vi "UDT__loggingModule_sendErrorLog.vi"() -> (3 "Unit Test Framework Results":T1)   [LabVIEW 2017]
doc: "Use this template to create a user-defined test VI. Define your test requirements and wire the results to the <b>Result (Test)</b> control. Do not modify the <b>Unit Test Framework Results</b> indicator."
uses:
  <vilib>/utf/common/utf_test_result_troll.ctl
  <vilib>/utf/common/utf_test_result.ctl
  <vilib>/utf/common/utf_test_result_failure.ctl
  <vilib>/utf/common/utf_test_comparison_operators.ctl
  <vilib>/utf/common/utf_vi_tag.ctl
  RT/loggingModule/Queue/TypeDefs/queueFGVState.ctl
  RT/ErrorMonitor/Queue/TypeDefs/message.ctl
  RT/loggingModule/loggingModule.lvlib
  <vilib>/Control Software Solutions Ltd/UTF Helper/Unit Test Helper.lvlib
  RT/ErrorMonitor/ErrorMonitor.lvlib
  <vilib>/utf/NI_UnitTestFramework.lvlib
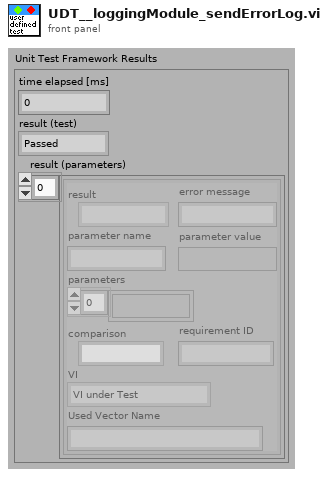
[diagram p1: front panel]
types:
  T1 = typedef "NI_UnitTestFramework.lvlib/utf_test_result_troll.ctl" = cluster{"time elapsed [ms]":u32, "result (test)":T2, "result (parameters)":T3[]}
  T2 = typedef "NI_UnitTestFramework.lvlib/utf_test_result.ctl" = enum16{"Passed", "Failed", "Error", "Skipped", "Not Processed"}
  T3 = typedef "NI_UnitTestFramework.lvlib/utf_test_result_failure.ctl" = cluster{"result":T2, "error message":string, "parameter name":string, "parameter value":variant, "parameters":variant[], "comparison":T4, "requirement ID":string, "VI":T5, "Used Vector Name":string}
  T4 = typedef "NI_UnitTestFramework.lvlib/utf_test_comparison_operators.ctl" = enum16{"=", "!=", ">", ">=", "<", "<=", "range", "symmetric tolerance", "asymmetric tolerance", "string contains", "string not contain", "array size", "string length", "array range", "by element", "array range (limit array)", "user-defined", "array contains", "array not contain", "vector length", "= (elm)", "!= (elm)", "= (case insensitive)", "!= (case insensitive)"}
  T5 = typedef "NI_UnitTestFramework.lvlib/utf_vi_tag.ctl" = enum16{"Setup VI", "VI under Test", "Teardown VI"}
  T6 = typedef "ErrorMonitor.lvlib/message.ctl" = cluster{"calling module":string, "message":string, "Data":variant}
  T7 = typedef "loggingModule.lvlib/queueFGVState.ctl" = enum16{"obtain", "enqueue low priority", "enqueue high priority", "dequeue", "release"}
  T8 = typedef "loggingModule.lvlib/message.ctl" = cluster{"calling module":string, "message":string, "data":variant}
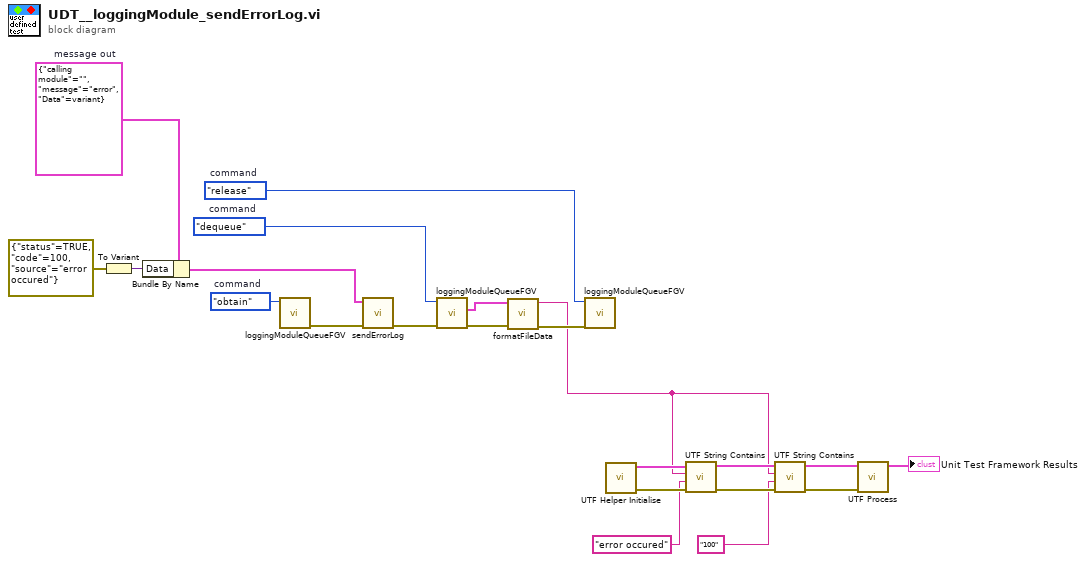
[diagram p0: block diagram]
diagram:
  w4 = T6 {"calling module"="", "message"="error", "Data"=variant}  # message out
  w20 = queueFGVState."release"  # command
  w21 = queueFGVState."dequeue"  # command
  w22 = queueFGVState."obtain"  # command
  n1 = To Variant(anything=errorcluster {"status"=TRUE, "code"=100, "source"="error occured"} ("error constant")) -> (Variant=w1:variant)
  n2 = Bundle By Name(cluster=w4, "Data"=w1) -> (w3:T6)
  n3 = call "loggingModuleQueueFGV.vi"("command"=w22) -> ("error out"=w6:errorcluster)  [unwired: 9 in, 1 out]
  n4 = call "sendErrorLog.vi"("error in (no error)"=w6, "message out"=w3) -> ("error out"=w5:errorcluster)  [unwired: 9 in]
  n5 = call "loggingModuleQueueFGV.vi"("error in (no error)"=w5, "command"=w21) -> ("error out"=w13:errorcluster, "message out"=w11:T8)  [unwired: 8 in]
  n6 = call "formatFileData.vi"("error in (no error)"=w13, "message out"=w11) -> ("error out"=w12:errorcluster, "LogData"=w10:string)  [unwired: 8 in]
  n7 = call "loggingModuleQueueFGV.vi"("error in (no error)"=w12, "command"=w20) -> ()  [unwired: 8 in, 2 out]
  n8 = call <vilib>:"UTF Helper Initialise.vi"() -> ("error out"=w14:errorcluster, "results array"=w15:T3[])  [unwired: 10 in]
  n9 = call <vilib>:"UTF String Contains.vi"("error in (no error)"=w14, "Test Value"="error occured", "Input"=w10, "Input Results"=w15) -> ("error out"=w16:errorcluster, "Output Results"=w17:T3[])  [unwired: 6 in]
  n10 = call <vilib>:"UTF String Contains.vi"("error in (no error)"=w16, "Test Value"="100", "Input"=w10, "Input Results"=w17) -> ("error out"=w19:errorcluster, "Output Results"=w18:T3[])  [unwired: 6 in]
  n11 = call <vilib>:"UTF Process.vi"("error in (no error)"=w19, "results array"=w18) -> ("Unit Test Framework Results"=→"Unit Test Framework Results":T1)  [unwired: 9 in]
